vi "Stop Acquisition.vi"(8 "error in (no error)":errorcluster caption="entrée d'erreur (pas d'erreur)", 10 "Session In":T1, 11 "Acq Cam Basler en entrée":refnum<class "Acq Cam Basler.lvclass">) -> (0 "error out":errorcluster caption="sortie d'erreur", 3 "Acq Cam Basler en sortie":refnum<class "Acq Cam Basler.lvclass">)   [LabVIEW 2023, in "Acq Cam Basler.lvclass"]
uses:
  Acq Cam Basler.lvclass
  <vilib>/userDefined/High Color/IMAQdx.ctl
  Acq Cam Basler.lvclass/Acq Cam Basler.ctl
  <vilib>/vision/driver/NI_Vision_Acquisition_Software.lvlib
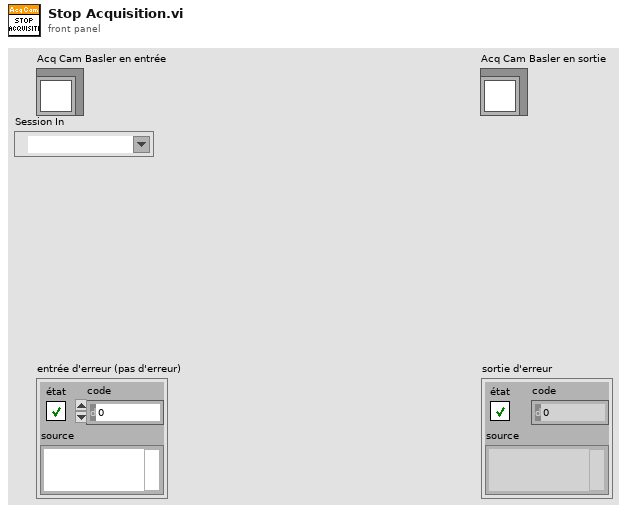
[diagram p1: front panel]
types:
  T1 = typedef "IMAQdx.ctl" = refnum<k21>
  T2 = typedef "IMAQ Image.ctl" = refnum<image>
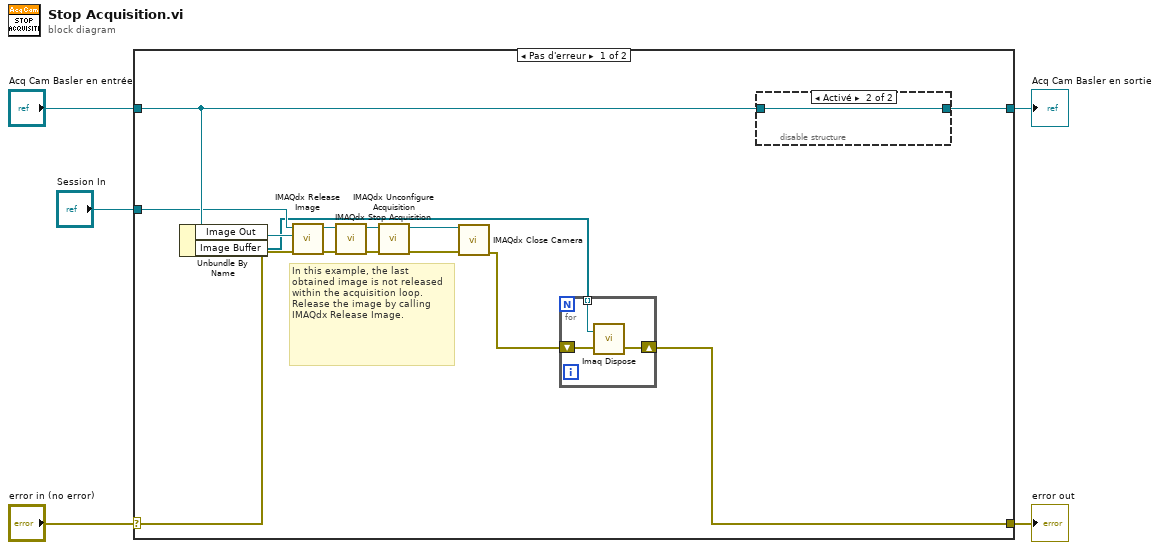
[diagram p0: block diagram]
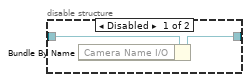
[diagram p2: hidden frame]
diagram:
  n1 = case shown="Pas d'erreur" "error in (no error)" {
    selector: "error in (no error)" -> [w15 w27]
    tunnel: [w7 w27] -> w4
    tunnel: [w14 w26] -> w2
    tunnel: "Acq Cam Basler en entrée" -> [w13 w26]
    tunnel: "Session In" -> [w11 _]
    frame No Error {
      # "In this example, the last obtained image is not released within the acquisition loop. Release the image by calling IMAQdx Release Image."
      n2 = Unbundle By Name(w13) -> ("Image Out"=w12:T2, "Image Buffer"=w6:T2[])
      n3 = call <vilib>:"IMAQdx Release Image.vi"("error in"=w15, "Image"=w12, "Session In"=w11) -> ("error out"=w17:errorcluster, "Session Out"=w16:T1)  [unwired: 7 in]
      n4 = call <vilib>:"IMAQdx Stop Acquisition.vi"("error in"=w17, "Session In"=w16) -> ("error out"=w18:errorcluster, "Session Out"=w19:T1)  [unwired: 8 out]
      n5 = call <vilib>:"IMAQdx Unconfigure Acquisition.vi"("error in"=w18, "Session In"=w19) -> ("error out"=w10:errorcluster, "Session Out"=w9:T1)  [unwired: 8 out]
      n6 = call <vilib>:"IMAQdx Close Camera.vi"("error in"=w10, "Session In"=w9) -> ("error out"=w8:errorcluster)  [unwired: 9 out]
      n7 = for {
        shift-right: [w24] -> w7
        shift-left: w8 -> [w25]
        tunnel: w6 -> [w23] mode=indexing
        n8 = call "Imaq Dispose"("Image"=w23, "error in (no error)"=w25) -> ("error out"=w24:errorcluster)  [unwired: 4 in]
      }
      n9 = disable-structure shown="Activé" {
        disable-tunnel: [w21 w22] -> w14
        disable-tunnel: w13 -> [w20 w22]
        frame Disabled {
          n10 = Bundle By Name(cluster=w20) -> (w21:refnum<class "Acq Cam Basler.lvclass">)  [unwired: 1 in]
        }
        frame Enabled {
        }
      }
    }
    frame Error {
    }
  }
  "error out" <- w4
  "Acq Cam Basler en sortie" <- w2
